vi "CRYPEAQ M1M2.vi"(10 "Model":u16(ring) items=["FFT", "Other"], 11 "Version":u16(ring) items=["Basic", "Advance", "Default"]) -> (2 "M2":dbl, 3 "M1":dbl)   [LabVIEW 2013]
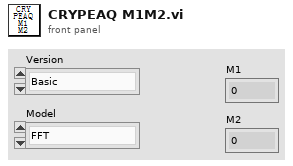
[diagram p1: front panel]
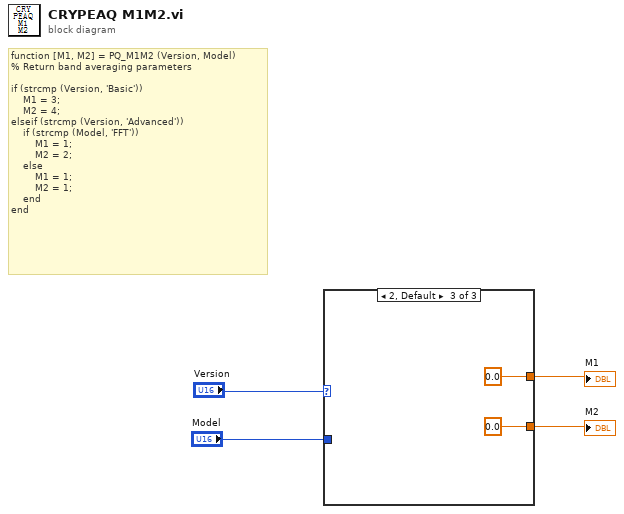
[diagram p0: block diagram]
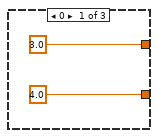
[diagram p2: hidden frame]
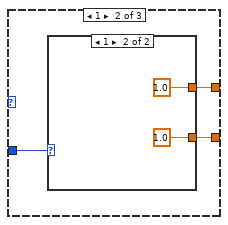
[diagram p3: hidden frame]
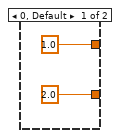
[diagram p4: hidden frame]
diagram:
  # "function [M1, M2] = PQ_M1M2 (Version, Model)\n% Return band averaging parameters\n\nif (strcmp (Version, 'Basic'))\n    M1 = 3;\n    M2 = 4;\nelseif (strcmp (Version, 'Advanced'))\n    if (strcmp (Model, 'FFT'))\n        M1 = 1;\n        M2 = 2;\n    else\n        M1 = 1;\n        M2 = 1;\n    end\nend"
  n1 = case shown="2, Default" "Version" {
    tunnel: [3.0 w9 0.0] -> w3
    tunnel: [4.0 w8 0.0] -> w2
    tunnel: "Model" -> [_ w7 _]
    frame 0 {
    }
    frame 1 {
      n2 = case shown="1" w7 {
        tunnel: [1.0 1.0] -> w9
        tunnel: [2.0 1.0] -> w8
        frame 0, Default {
        }
        frame 1 {
        }
      }
    }
    frame 2, Default {
    }
  }
  "M1" <- w3
  "M2" <- w2
